vi "CRYASIO Play & Receive.vi"(10 "ASIO Play Cluster In":T2(array[cluster]), 11 "ASIO Record Cluster In":T1(array[cluster])) -> (3 "ASIO Record Cluster Out":T1(array[cluster]))   [LabVIEW 2013]
uses:
  CRYMainGlobal.vi
  Task Sequence/CRYProject Run Control Global.vi
  CRYAcquisition Global.vi
panel:
  out "bResult":bool
  out "Buff Index Array":i32[](array[numeric])
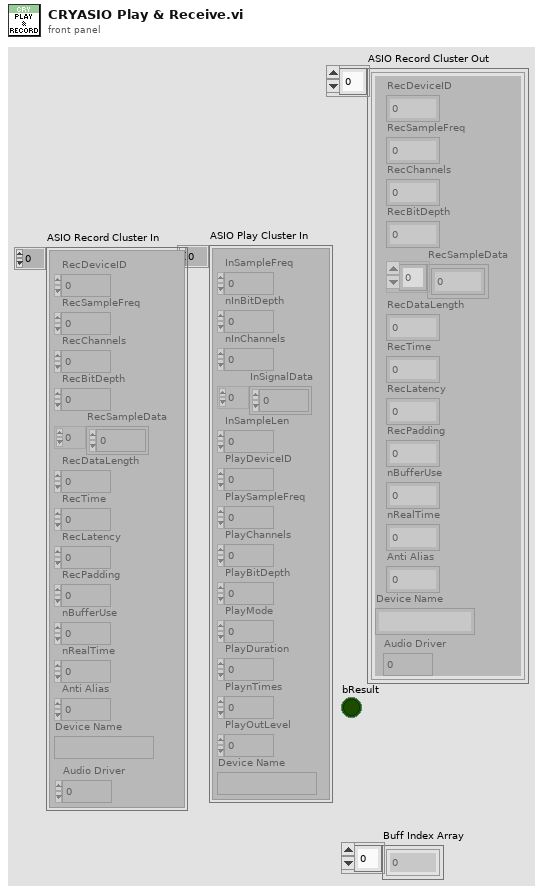
[diagram p1: front panel]
types:
  T1 = cluster{"RecDeviceID":u32, "RecSampleFreq":u32, "RecChannels":u32, "RecBitDepth":u32, "RecSampleData":i32[], "RecDataLength":u32, "RecTime":sgl, "RecLatency":sgl, "RecPadding":sgl, "nBufferUse":u32, "nRealTime":u32, "Anti Alias":u32, "Device Name":string, "Audio Driver":u16}[]
  T2 = cluster{"InSampleFreq":u32, "nInBitDepth":u32, "nInChannels":u32, "InSignalData":sgl[], "InSampleLen":u32, "PlayDeviceID":u32, "PlaySampleFreq":u32, "PlayChannels":u32, "PlayBitDepth":u32, "PlayMode":u32, "PlayDuration":sgl, "PlaynTimes":u32, "PlayOutLevel":sgl, "Device Name":string}[]
  T3 = cluster{"RecDeviceID":u32, "RecSampleFreq":u32, "RecChannels":u32, "RecBitDepth":u32, "RecSampleData":i32[], "RecDataLength":u32, "RecTime":sgl, "RecLatency":sgl, "RecPadding":sgl, "nBufferUse":u32, "nRealTime":u32, "Anti Alias":u32, "Device Name":string, "Audio Driver":u16}
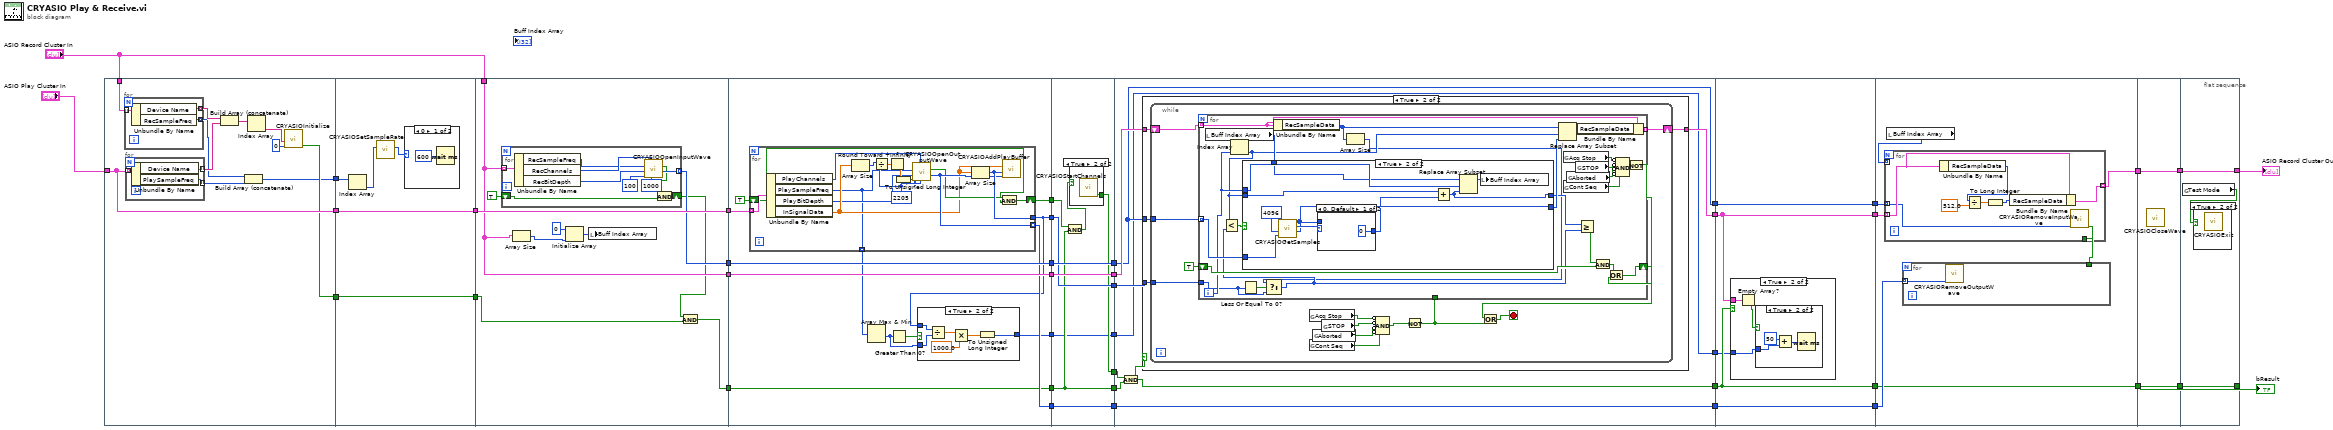
[diagram p0: block diagram]
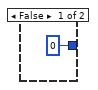
[diagram p3: hidden frame]
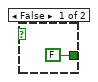
[diagram p4: hidden frame]
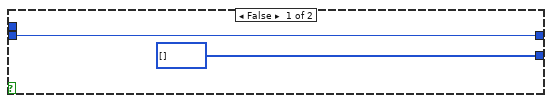
[diagram p6: hidden frame]
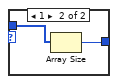
[diagram p7: hidden frame]
diagram:
  n1 = flat-sequence {
    tunnel: [w51] -> w18
    tunnel: "ASIO Record Cluster In" -> [w50]
    tunnel: [w44] -> w16
    tunnel: "ASIO Play Cluster In" -> [w51]
    tunnel: [w41] -> w14
    tunnel: w18 -> [w62]
    tunnel: [w62] -> w17
    tunnel: w16 -> [w61]
    tunnel: [w61] -> w15
    tunnel: w14 -> [w60]
    tunnel: "ASIO Record Cluster In" -> [w70]
    tunnel: [w73] -> w39
    tunnel: w17 -> [w73]
    tunnel: [w70] -> w38
    tunnel: [w72] -> w35
    tunnel: [w64] -> w25
    tunnel: w15 -> [w65]
    tunnel: w39 -> [w93]
    tunnel: w38 -> [w95]
    tunnel: [w95] -> w36
    tunnel: w35 -> [w94]
    tunnel: [w94] -> w33
    tunnel: [w86] -> w32
    tunnel: [w92] -> w27
    tunnel: w25 -> [w91]
    tunnel: [w91] -> w23
    tunnel: [w89] -> w22
    tunnel: [w84] -> w2
    tunnel: [w126] -> w37
    tunnel: w36 -> [w126]
    tunnel: [w125] -> w34
    tunnel: w33 -> [w125]
    tunnel: w32 -> [w124]
    tunnel: [w124] -> w31
    tunnel: w27 -> [w123]
    tunnel: [w123] -> w26
    tunnel: [w121] -> w24
    tunnel: w23 -> [w121]
    tunnel: w22 -> [w122]
    tunnel: [w119] -> w21
    tunnel: w2 -> [w118]
    tunnel: [w118] -> w1
    tunnel: w37 -> [w137]
    tunnel: w34 -> [w135]
    tunnel: w31 -> [w130]
    tunnel: [w136] -> w11
    tunnel: [w135] -> w9
    tunnel: [w134] -> w7
    tunnel: w26 -> [w134]
    tunnel: w24 -> [w133]
    tunnel: w21 -> [w132]
    tunnel: [w131] -> w5
    tunnel: [w129] -> w3
    tunnel: w1 -> [w129]
    tunnel: w11 -> [w197]
    tunnel: [w197] -> w10
    tunnel: w9 -> [w200]
    tunnel: [w200] -> w8
    tunnel: w7 -> [w199]
    tunnel: [w199] -> w6
    tunnel: w5 -> [w198]
    tunnel: [w198] -> w4
    tunnel: w3 -> [w196]
    tunnel: [w212] -> w30
    tunnel: w10 -> [w211]
    tunnel: w8 -> [w209]
    tunnel: w6 -> [w208]
    tunnel: [w207] -> w20
    tunnel: w4 -> [w207]
    tunnel: w30 -> [w224]
    tunnel: w20 -> [w223]
    tunnel: [w224] -> w13
    tunnel: [w223] -> w12
    tunnel: [w226] -> w19
    tunnel: [w227] -> w29
    tunnel: w13 -> [w227]
    tunnel: w12 -> [w226]
    frame #0 {
      n2 = for {
        tunnel: [w53] -> _ mode=indexing
        tunnel: [w54] -> w49 mode=indexing
        tunnel: w50 -> [w53] mode=indexing
        tunnel: [w52] -> w43 mode=indexing
        n3 = Unbundle By Name(w53) -> ("Device Name"=w54:string, "RecSampleFreq"=w52:u32)
      }
      n4 = for {
        tunnel: w51 -> [w57] mode=indexing
        tunnel: [w56] -> w48 mode=indexing
        tunnel: [w55] -> w42 mode=indexing
        n5 = Unbundle By Name(w57) -> ("Device Name"=w56:string, "PlaySampleFreq"=w55:u32)
      }
      n6 = Build Array (concatenate)(w49, w48) -> (w47:string[])
      n7 = Build Array (concatenate)(w43, w42) -> (w41:u32[])
      n8 = Index Array(array=w47) -> (element=w46:string)  [unwired: 1 in]
      n9 = call "CRYASIOInitialize.vi"("Sampling Rate"=u32 0, "Driver Name"=w46) -> ("bResult"=w44:bool)  [unwired: 8 in, 1 out]
    }
    frame #1 {
      n10 = Index Array(array=w60) -> (element=w59:u32)  [unwired: 1 in]
      n11 = call "CRYASIOSetSampleRate.vi"("fs"=w59) -> ("return type"=w58:i32)  [unwired: 9 in, 1 out]
      n12 = case shown="0" w58 {
        frame 0 {
          n13 = Wait (ms)(milliseconds to wait=u32 600) -> ()  [unwired: 1 out]
        }
        frame 1, Default {
        }
      }
    }
    frame #2 {
      n14 = for {
        tunnel: w70 -> [w83] mode=indexing
        tunnel: [w77] -> w72 mode=indexing
        shift-right: [w75] -> w66
        shift-left: TRUE -> [w74]
        n15 = Unbundle By Name(w83) -> ("RecSampleFreq"=w81:u32, "RecChannels"=w82:u32, "RecBitDepth"=w80:u32)
        n16 = call "CRYASIOOpenInputWave.vi"("Buff Length"=u32 1000 ("Wave Length"), "Channel Index"=w82, "Buff Count"=u32 100 ("Unknown"), "Bit Depth"=w80, "Sampling Rate"=w81) -> ("Opend Channel Index"=w77:u32, "bResult"=w76:bool)  [unwired: 3 in, 1 out]
        n17 = And(x=w76, y=w74) -> (x .and. y?=w75:bool)
      }
      n18 = Array Size(array=w70) -> (size(s)=w69:i32)
      n19 = Initialize Array(0 ("element"), w69) -> (w68:i32[])
      n20 = local write "Buff Index Array"(w68) -> ()
      n21 = And(x=w66, y=w65) -> (x .and. y?=w64:bool)
    }
    frame #3 {
      n22 = for {
        tunnel: w93 -> [w116] mode=indexing
        tunnel: [w115] -> w86
        tunnel: [w109] -> w92 mode=indexing
        shift-right: [w107] -> w89
        shift-left: TRUE -> [w106]
        tunnel: [w103] -> w88 mode=indexing
        w113 = u32 2205 ("Wave Length")
        n23 = Unbundle By Name(w116) -> ("PlayChannels"=w117:u32, "PlaySampleFreq"=w103:u32, "PlayBitDepth"=w104:u32, "InSignalData"=w105:sgl[])
        n24 = Array Size(array=w105) -> (size(s)=w114:i32)
        n25 = Divide(x=w114, y=w113) -> (x/y=w112:dbl)
        n26 = Round Toward +Infinity(x=w112) -> (ceil(x): smallest int >= x=w110:dbl)
        n27 = To Unsigned Long Integer(number=w110) -> (unsigned 32bit integer=w111:u32)
        n28 = call "CRYASIOOpenOutputWave.vi"("Buff Length"=w113, "Channel Index"=w117, "Buff Count"=w111, "Bit Depth"=w104, "Sampling Rate"=w103) -> ("OCI"=w109:u32, "bResult"=w108:bool)  [unwired: 3 in, 1 out]
        n29 = Array Size(array=w105) -> (size(s)=w115:i32)
        n30 = And(x=w108, y=w106) -> (x .and. y?=w107:bool)
        n31 = call "CRYASIOAddPlayBuffer.vi"("Limit"=w109, "Data Length"=w115, "pData"=w105) -> ()  [unwired: 5 in, 3 out]
      }
      n32 = Array Max & Min(array=w88) -> (min value=w85:u32)  [unwired: 3 out]
      n33 = Greater Than 0?(x=w85) -> (x > 0?=w87:bool)
      n34 = case shown="True" w87 {
        tunnel: w86 -> [_ w102]
        tunnel: w85 -> [_ w101]
        tunnel: [0 w97] -> w84
        frame False {
        }
        frame True {
          n35 = Divide(x=w102, y=w101) -> (x/y=w100:dbl)
          n36 = Multiply(x=w100, y=1000.0) -> (x*y=w98:dbl)
          n37 = To Unsigned Long Integer(number=w98) -> (unsigned 32bit integer=w97:u32)
        }
      }
    }
    frame #4 {
      n38 = And(x=w122, y=w121) -> (x .and. y?=w120:bool)
      n39 = case shown="True" w120 {
        tunnel: [FALSE ("bResult") w128] -> w119
        frame False {
        }
        frame True {
          n40 = call "CRYASIOStartChannels.vi"() -> ("bResult"=w128:bool)  [unwired: 10 in, 1 out]
        }
      }
    }
    frame #5 {
      n41 = And(x=w132, y=w133) -> (x .and. y?=w131:bool)
      n42 = case shown="True" w131 {
        tunnel: w130 -> [_ w142]
        tunnel: w137 -> [w138 w141]
        tunnel: [w138 w140] -> w136
        tunnel: w135 -> [_ w139]
        frame False {
        }
        frame True {
          n43 = while {
            tunnel: w139 -> [w155]
            tunnel: w142 -> [w154]
            shift-right: [w143] -> w140
            shift-left: w141 -> [w144]
            stop <- w146 stop-if-true
            n44 = global read "CRYMainGlobal.vi" "Acq Stop"() -> (w152:bool)
            n45 = global read "CRYProject Run Control Global.vi" "Cont Seq"() -> (w149:bool)
            n46 = global read "CRYProject Run Control Global.vi" "Aborted"() -> (w150:bool)
            n47 = global read "CRYMainGlobal.vi" "STOP"() -> (w151:bool)
            n48 = Compound Arithmetic op=AND(invert w152, invert w151, invert w150, invert w149) -> (w148:bool)
            n49 = Not(x=w148) -> (.not. x?=w145:bool)
            n50 = for {
              tunnel: w155 -> [w177] mode=indexing
              tunnel: w154 -> [w159]
              shift-right: [w170] -> w147
              shift-left: TRUE -> [w179]
              tunnel: w145 -> [_]
              tunnel: w144 -> [w174] mode=indexing
              tunnel: [w171] -> w143 mode=indexing
              i -> [w176]
              n51 = local read "Buff Index Array"() -> (w162:i32[])
              n52 = Index Array(array=w162, index=w176) -> (element=w161:i32)
              n53 = Less Or Equal To 0?(x=w159) -> (x <= 0?=w160:bool)
              n54 = Unbundle By Name(w174) -> ("RecSampleData"=w157:i32[])
              n55 = Array Size(array=w157) -> (size(s)=w156:i32)
              n56 = Select(t=w156, s=w160, f=w159) -> (s? t:f=w158:i32)
              n57 = Less?(x=w161, y=w158) -> (x < y?=w178:bool)
              n58 = case shown="True" w178 {
                tunnel: w177 -> [_ w192]
                tunnel: [i32[] [] ("pData") w186] -> w175
                tunnel: w176 -> [_ w190]
                tunnel: [w181 w189] -> w172
                tunnel: w162 -> [_ w184]
                tunnel: w161 -> [w181 w183]
                frame False {
                }
                frame True {
                  n59 = call "CRYASIOGetSamples.vi"("Limit"=w192, "Data Length"=4096 ("y")) -> ("pData"=w186:i32[], "nResult"=w188:u32)  [unwired: 5 in, 2 out]
                  n60 = case shown="0, Default" w188 {
                    tunnel: w186 -> [_ w195]
                    tunnel: [0 w194] -> w185
                    frame 0, Default {
                    }
                    frame 1 {
                      n61 = Array Size(array=w195) -> (size(s)=w194:i32)
                    }
                  }
                  n62 = Add(x=w183, y=w185) -> (x+y=w189:i32)
                  n63 = Replace Array Subset(array=w184, new element=w189, index=w190) -> (w191:i32[])
                  n64 = local write "Buff Index Array"(w191) -> ()
                }
              }
              n65 = Replace Array Subset(array=w157, new element=w175, index=w161) -> (w173:i32[])
              n66 = global read "CRYMainGlobal.vi" "Acq Stop"() -> (w169:bool)
              n67 = global read "CRYProject Run Control Global.vi" "Cont Seq"() -> (w166:bool)
              n68 = global read "CRYProject Run Control Global.vi" "Aborted"() -> (w167:bool)
              n69 = global read "CRYMainGlobal.vi" "STOP"() -> (w168:bool)
              n70 = Bundle By Name(cluster=w174, "RecSampleData"=w173) -> (w171:T3)
              n71 = Greater Or Equal?(x=w172, y=w158) -> (x >= y?=w180:bool)
              n72 = And(x=w180, y=w179) -> (x .and. y?=w164:bool)
              n73 = Compound Arithmetic op=AND(invert w169, invert w168, invert w167, invert w166) -> (w165:bool)
              n74 = Not(x=w165) -> (.not. x?=w163:bool)
              n75 = Or(x=w164, y=w163) -> (x .or. y?=w170:bool)
            }
            n76 = Or(x=w147, y=w145) -> (x .or. y?=w146:bool)
          }
        }
      }
    }
    frame #6 {
      n77 = case shown="True" w198 {
        tunnel: w197 -> [_ w203]
        tunnel: w196 -> [_ w201]
        frame False {
        }
        frame True {
          n78 = Empty Array?(array=w203) -> (empty?=w202:bool)
          n79 = case shown="True" w202 {
            tunnel: w201 -> [_ w206]
            frame False {
            }
            frame True {
              n80 = Add(x=u32 50, y=w206) -> (x+y=w204:u32)
              n81 = Wait (ms)(milliseconds to wait=w204) -> ()  [unwired: 1 out]
            }
          }
        }
      }
    }
    frame #7 {
      n82 = local read "Buff Index Array"() -> (w210:i32[])
      n83 = for {
        tunnel: w211 -> [w221] mode=indexing
        tunnel: [w222] -> w213
        tunnel: [w220] -> w212 mode=indexing
        tunnel: w210 -> [_] mode=indexing
        tunnel: w209 -> [w219] mode=indexing
        n84 = Unbundle By Name(w221) -> ("RecSampleData"=w216:i32[])
        n85 = Divide(x=w216, y=512.0) -> (x/y=w217:dbl[])
        n86 = To Long Integer(number=w217) -> (32bit integer=w215:i32[])
        n87 = Bundle By Name(cluster=w221, "RecSampleData"=w215) -> (w220:T3)
        n88 = call "CRYASIORemoveInputWave.vi"("OCI"=w219) -> ("bResult"=w222:bool)  [unwired: 9 in, 1 out]
      }
      n89 = for {
        tunnel: w213 -> [_]
        tunnel: w208 -> [w214] mode=indexing
        n90 = call "CRYASIORemoveOutputWave.vi"("OCI"=w214) -> ()  [unwired: 9 in, 2 out]
      }
    }
    frame #8 {
      n91 = call "CRYASIOCloseWave.vi"() -> ()  [unwired: 10 in, 2 out]
    }
    frame #9 {
      n92 = global read "CRYAcquisition Global.vi" "Test Mode"() -> (w225:bool)
      n93 = case shown="True" w225 {
        frame False {
        }
        frame True {
          n94 = call "CRYASIOExit.vi"() -> ()  [unwired: 10 in, 2 out]
        }
      }
    }
  }
  "ASIO Record Cluster Out" <- w29
  "bResult" <- w19
